vi "rsscope_core_global.vi"() -> ()   [LabVIEW 2014] (continued)
"Descriptive Name"="Trigger Event Beep", "Data Type"=0, "Command"="TRIG:EVEN:BEEP", "Access"=2, "Range Table"="RsScope_rngTriggerEvent", "Read Callback"="", "Write Callback"="", "Supported Models"="", "Instrument Options"="", "Flags"=0, "Help"="Generates a beep sound if the command is set to trigger.\n\nAvailable Repeated Capabilities:\nNone\n\nRemote-control command(s):\nTRIGger<m>:EVENt:BEEP"}, {"Level"=2, "Class Only"=FALSE, "Identifier"="RSSCOPE_ATTR_TRIGGER_EVENT_PRINT", "Descriptive Name"="Trigger Event Print", "Data Type"=0, "Command"="TRIG:EVEN:PRIN", "Access"=2, "Range Table"="RsScope_rngTriggerEvent", "Read Callback"="", "Write Callback"="", "Supported Models"="", "Instrument Options"="", "Flags"=0, "Help"="Saves a screenshot at each trigger if the command is set to trigger.\n\nAvailable Repeated Capabilities:\nNone\n\nRemote-control command(s):\nTRIGger<m>:EVENt:PRINt"}, {"Level"=2, "Class Only"=FALSE, "Identifier"="RSSCOPE_ATTR_TRIGGER_EVENT_SAVE_WAVEFORM", "Descriptive Name"="Trigger Event Save Waveform", "Data Type"=0, "Command"="TRIG:EVEN:WFMS", "Access"=2, "Range Table"="RsScope_rngTriggerEvent", "Read Callback"="", "Write Callback"="", "Supported Models"="", "Instrument Options"="", "Flags"=0, "Help"="Saves the waveform data to file at each trigger if the command is set to trigger.\n\nAvailable Repeated Capabilities:\nNone\n\nRemote-control command(s):\nTRIGger<m>:EVENt:WFMSave"}, {"Level"=2, "Class Only"=FALSE, "Identifier"="RSSCOPE_ATTR_TRIGGER_EVENT_RUN_EXTERNAL_APPLICATION", "Descriptive Name"="Trigger Event Run External Application", "Data Type"=0, "Command"="TRIG:EVEN:RUN", "Access"=2, "Range Table"="RsScope_rngTriggerEvent", "Read Callback"="", "Write Callback"="", "Supported Models"="", "Instrument Options"="", "Flags"=0, "Help"="Starts an external application if the attribute is set to trigger.\nUse the following attributes to set up the application:\nRSSCOPE_ATTR_EXTERNAL_APPLICATION_NAME\nRSSCOPE_ATTR_EXTERNAL_APPLICATION_PARAMETER\nRSSCOPE_ATTR_EXTERNAL_APPLICATION_WORKING_DIRECTORY\n\nAvailable Repeated Capabilities:\nNone\n\nRemote-control command(s):\nTRIGger<m>:EVENt:RUNexec"}, {"Level"=2, "Class Only"=FALSE, "Identifier"="RSSCOPE_ATTR_TRIGGER_EXTERNAL_OVERLOAD", "Descriptive Name"="Trigger External Overload", "Data Type"=3, "Command"="TRIG{Trigger}:EXT:OVER", "Access"=2, "Range Table"="", "Read Callback"="", "Write Callback"="", "Supported Models"="", "Instrument Options"="", "Flags"=0, "Help"="Sets the overload status of the external trigger input.\n\nAvailable Repeated Capabilities:\nTrigger: TrigA, TrigB, TrigR\r\n\nRemote-control command(s):\nTRIGger<m>:EXTern:OVERload"}, {"Level"=2, "Class Only"=FALSE, "Identifier"="RSSCOPE_ATTR_DIGITAL_FILTER_TRIGGER_COUPLING", "Descriptive Name"="Digital Filter Trigger Coupling", "Data Type"=0, "Command"="TRIG{Trigger}:COUP", "Access"=2, "Range Table"="rsscope_rngDSPTriggCoupling", "Read Callback"="", "Write Callback"="", "Supported Models"="", "Instrument Options"="", "Flags"=0, "Help"="Selects the filter for the trigger channel(s). Other channels must use the same filter, or proceed unfiltered.\n\nAvailable Repeated Capabilities:\nTrigger: TrigA, TrigB, TrigR\r\n\nRemote-control command(s):\nTRIGger<m>:COUPling"}, {"Level"=2, "Class Only"=FALSE, "Identifier"="RSSCOPE_ATTR_HIGH_FREQUENCY_REJECT_TRIGGER_STATE", "Descriptive Name"="High Frequency Reject Trigger State", "Data Type"=3, "Command"="TRIG{Trigger}:RFSR", "Access"=2, "Range Table"="", "Read Callback"="", "Write Callback"="", "Supported Models"="RTE", "Instrument Options"="", "Flags"=0, "Help"="Enables the DSP filter for the trigger channel. Frequencies higher than the bandwidth (RSSCOPE_ATTR_DIGITAL_FILTER_TRIGGER_RF_REJECT) are rejected, lower frequencies pass the filter.\n\nAvailable Repeated Capabilities:\nTrigger: TrigA, TrigB, TrigR\r\n\nRemote-control command(s):\nTRIGger<m>:RFSReject"}, {"Level"=2, "Class Only"=FALSE, "Identifier"="RSSCOPE_ATTR_TRIGGER_AC_POWER_INPUT_SLOPE", "Descriptive Name"="Trigger AC Power Input Slope", "Data Type"=0, "Command"="TRIG{Trigger}:POW:SLOP", "Access"=2, "Range Table"="rsscope_rngTriggerACPowerInputSlope", "Read Callback"="", "Write Callback"="", "Supported Models"="RTE", "Instrument Options"="", "Flags"=0, "Help"="Selects the rising or falling edges of the AC power input for the trigger condition.\n\nAvailable Repeated Capabilities:\nTrigger: TrigA, TrigB, TrigR\r\n\nRemote-control command(s):\nTRIGger<m>:POWerline:SLOPe"}, {"Level"=2, "Class Only"=TRUE, "Identifier"="", "Descriptive Name"="Channel", "Data Type"=0, "Command"="", "Access"=0, "Range Table"="", "Read Callback"="", "Write Callback"="", "Supported Models"="", "Instrument Options"="", "Flags"=0, "Help"="Indicates the trigger source channel"}, {"Level"=3, "Class Only"=FALSE, "Identifier"="RSSCOPE_ATTR_TRIGGER_LEVEL", "Descriptive Name"="Trigger Level", "Data Type"=1, "Command"="TRIG{Trigger}:LEV{TriggerSource}", "Access"=2, "Range Table"="", "Read Callback"="", "Write Callback"="", "Supported Models"="", "Instrument Options"="", "Flags"=0, "Help"="Sets the trigger level for the specified event and source.\n\nAvailable Repeated Capabilities:\nTrigger: TrigA, TrigB, TrigR\r\nTriggerSource: TsCH1, TsCH2, TsCH3, TsCH4, TsExt, TsLine, TsZ1V1, TsZ1V2, TsZ1V3, TsZ1V4, TsZ1I1, TsZ1I2, TsZ1I3, TsZ1I4, TsZ2V1, TsZ2V2, TsZ2V3, TsZ2V4, TsZ2I1, TsZ2I2, TsZ2I3, TsZ2I4, TsDiff1, TsDiff2, TsCommon1, TsCommon2\r\n\nRemote-control command(s):\nTRIGger<m>:LEVel<n>[:VALue]"}, {"Level"=3, "Class Only"=FALSE, "Identifier"="RSSCOPE_ATTR_DIGITAL_FILTER_TRIGGER_RF_REJECT", "Descriptive Name"="Digital Filter Trigger RF Reject", "Data Type"=1, "Command"="TRIG{Trigger}:RFR", "Access"=2, "Range Table"="rsscope_rngDSPTriggRFReject", "Read Callback"="", "Write Callback"="", "Supported Models"="", "Instrument Options"="", "Flags"=0, "Help"="Sets the limit frequency, if the trigger coupling is set to RFReject. See RSSCOPE_ATTR_DIGITAL_FILTER_TRIGGER_COUPLING\n\nAvailable Repeated Capabilities:\nTrigger: TrigA, TrigB, TrigR\r\n\nRemote-control command(s):\nTRIGger<m>:RFReject"}, {"Level"=2, "Class Only"=TRUE, "Identifier"="", "Descriptive Name"="Edge Triggering", "Data Type"=0, "Command"="", "Access"=0, "Range Table"="", "Read Callback"="", "Write Callback"="", "Supported Models"="", "Instrument Options"="", "Flags"=0, "Help"="Attributes that configure the edge trigger.  An edge trigger occurs when the trigger signal passes through the voltage threshold you specify with the RSSCOPE_ATTR_TRIGGER_LEVEL attribute and has the slope you specify with the RSSCOPE_ATTR_TRIGGER_SLOPE attribute."}, {"Level"=3, "Class Only"=FALSE, "Identifier"="RSSCOPE_ATTR_EXTERNAL_TRIGGER_COUPLING", "Descriptive Name"="External Trigger Coupling", "Data Type"=0, "Command"="TRIG:ANED:COUP", "Access"=2, "Range Table"="rsscope_rngTriggerCoupling", "Read Callback"="", "Write Callback"="", "Supported Models"="", "Instrument Options"="", "Flags"=0, "Help"="Sets the coupling for the analog trigger signal.\n\nAvailable Repeated Capabilities:\nNone\n\nRemote-control command(s):\nTRIGger<m>:ANEDge:COUPling"}, {"Level"=3, "Class Only"=FALSE, "Identifier"="RSSCOPE_ATTR_TRIGGER_SLOPE", "Descriptive Name"="Trigger Slope", "Data Type"=0, "Command"="TRIG{Trigger}:EDGE:SLOP", "Access"=2, "Range Table"="rsscope_rngTriggerSlope", "Read Callback"="", "Write Callback"="", "Supported Models"="", "Instrument Options"="", "Flags"=0, "Help"="Sets the slope for the edge trigger.\n\nAvailable Repeated Capabilities:\nTrigger: TrigA, TrigB, TrigR\r\n\nRemote-control command(s):\nTRIGger<m>:EDGE:SLOPe"}, {"Level"=3, "Class Only"=FALSE, "Identifier"="RSSCOPE_ATTR_EXTERNAL_TRIGGER_LEVEL", "Descriptive Name"="External Trigger Level", "Data Type"=1, "Command"="TRIG:LEV5", "Access"=2, "Range Table"="", "Read Callback"="", "Write Callback"="", "Supported Models"="", "Instrument Options"="", "Flags"=0, "Help"="Sets the trigger level for the analog external trigger input.\n\nAvailable Repeated Capabilities:\nNone\n\nRemote-control command(s):\nTRIGger<m>:LEVel<n>[:VALue]"}, {"Level"=3, "Class Only"=FALSE, "Identifier"="RSSCOPE_ATTR_EXTERNAL_TRIGGER_FILTER_CUT_OFF_FREQUENCY_HIGHPASS", "Descriptive Name"="External Trigger Filter Cut Off Frequency Highpass", "Data Type"=0, "Command"="TRIG:ANED:CUT:HIGH", "Access"=2, "Range Table"="rsscope_rngCutOffFrequency", "Read Callback"="", "Write Callback"="", "Supported Models"="", "Instrument Options"="", "Flags"=0, "Help"="Defines highpass &apos;Cut-off&apos; frequency of filter.\n\nAvailable Repeated Capabilities:\nNone\n\nRemote-control command(s):\nTRIGger<m>:ANEDge:CUToff:HIGHpass"}, {"Level"=3, "Class Only"=FALSE, "Identifier"="RSSCOPE_ATTR_EXTERNAL_TRIGGER_FILTER_CUT_OFF_FREQUENCY_LOWPASS", "Descriptive Name"="External Trigger Filter Cut Off Frequency Lowpass", "Data Type"=0, "Command"="TRIGger1:ANED:CUT:LOWP", "Access"=2, "Range Table"="rsscope_rngCutOffFrequency", "Read Callback"="", "Write Callback"="", "Supported Models"="", "Instrument Options"="", "Flags"=0, "Help"="Defines lowpass &apos;Cut-off&apos; frequency of filter.\n\nAvailable Repeated Capabilities:\nNone\n\nRemote-control command(s):\nTRIGger<m>:ANEDge:CUToff:LOWPass"}, {"Level"=3, "Class Only"=FALSE, "Identifier"="RSSCOPE_ATTR_EXTERNAL_TRIGGER_FILTER", "Descriptive Name"="External Trigger Filter", "Data Type"=0, "Command"="TRIG:ANED:FILT", "Access"=2, "Range Table"="rsscope_rngFilterType", "Read Callback"="", "Write Callback"="", "Supported Models"="", "Instrument Options"="", "Flags"=0, "Help"="The analog trigger signal is used for triggering; you can directly select an additional filter to reject high or low frequencies.\n\nAvailable Repeated Capabilities:\nNone\n\nRemote-control command(s):\nTRIGger<m>:ANEDge:FILTer"}, {"Level"=3, "Class Only"=FALSE, "Identifier"="RSSCOPE_ATTR_EXTERNAL_TRIGGER_GROUND_CONNECTION_ENABLED", "Descriptive Name"="External Trigger Ground Connection Enabled", "Data Type"=3, "Command"="TRIG:ANED:GND", "Access"=2, "Range Table"="", "Read Callback"="", "Write Callback"="", "Supported Models"="", "Instrument Options"="", "Flags"=0, "Help"="Connects the analog signal to the ground.\n\nAvailable Repeated Capabilities:\nNone\n\nRemote-control command(s):\nTRIGger<m>:ANEDge:GND"}, {"Level"=3, "Class Only"=FALSE, "Identifier"="RSSCOPE_ATTR_EXTERNAL_TRIGGER_SLOPE", "Descriptive Name"="External Trigger Slope", "Data Type"=0, "Command"="TRIG:ANED:SLOP", "Access"=2, "Range Table"="rsscope_rngPolarity", "Read Callback"="", "Write Callback"="", "Supported Models"="", "Instrument Options"="", "Flags"=0, "Help"="Sets the edge for the trigger event. Value 'Either' is not allowed.\n\nAvailable Repeated Capabilities:\nNone\n\nRemote-control command(s):\nTRIGger<m>:ANEDge:SLOPe"}, {"Level"=3, "Class Only"=FALSE, "Identifier"="RSSCOPE_ATTR_EXTERNAL_TRIGGER_NOISE_REJECT", "Descriptive Name"="External Trigger Noise Reject", "Data Type"=3, "Command"="TRIGger1:ANED:NREJ", "Access"=2, "Range Table"="", "Read Callback"="", "Write Callback"="", "Supported Models"="", "Instrument Options"="", "Flags"=0, "Help"="Enables/disbales the noise reject for the external trigger input.\n\nAvailable Repeated Capabilities:\nNone\n\nRemote-control command(s):\nTRIGger<m>:ANEDge:NREJect"}, {"Level"=2, "Class Only"=TRUE, "Identifier"="", "Descriptive Name"="Runt Triggering", "Data Type"=0, "Command"="", "Access"=0, "Range Table"="", "Read Callback"="", "Write Callback"="", "Supported Models"="", "Instrument Options"="", "Flags"=0, "Help"="A runt is a pulse lower than normal in amplitude. The amplitude crosses the first threshold twice in succession without crossing the second one. In addition to the threshold amplitudes, you can define a time limit for the runt in the same way as for width triggers. For example, this trigger can detect logic, digital, and analog signals remaining below a specified threshold amplitude because I/O ports are in undefined state."}, {"Level"=3, "Class Only"=FALSE, "Identifier"="RSSCOPE_ATTR_RUNT_CONDITION", "Descriptive Name"="Runt Condition", "Data Type"=0, "Command"="TRIG{Trigger}:RUNT:RANG", "Access"=2, "Range Table"="rsscope_rngRuntCondition", "Read Callback"="", "Write Callback"="", "Supported Models"="", "Instrument Options"="", "Flags"=0, "Help"="Defines the time limit of the runt pulse in relation to the TRIGger<m>: RUNT: WIDTh and TRIGger<m>: RUNT: DELTa settings.\n\nAvailable Repeated Capabilities:\nTrigger: TrigA, TrigB, TrigR\r\n\nRemote-control command(s):\nTRIGger<m>:RUNT:RANGe"}, {"Level"=3, "Class Only"=FALSE, "Identifier"="RSSCOPE_ATTR_RUNT_WIDTH", "Descriptive Name"="Runt Width", "Data Type"=1, "Command"="TRIG{Trigger}:RUNT:WIDT", "Access"=2, "Range Table"="rsscope_rngWidth", "Read Callback"="", "Write Callback"="", "Supported Models"="", "Instrument Options"="", "Flags"=0, "Help"="Defines the upper or lower voltage threshold.\n\nAvailable Repeated Capabilities:\nTrigger: TrigA, TrigB, TrigR\r\n\nRemote-control command(s):\nTRIGger<m>:RUNT:WIDTh"}, {"Level"=3, "Class Only"=FALSE, "Identifier"="RSSCOPE_ATTR_RUNT_DELTA", "Descriptive Name"="Runt Delta", "Data Type"=1, "Command"="TRIG{Trigger}:RUNT:DELT", "Access"=2, "Range Table"="", "Read Callback"="", "Write Callback"="", "Supported Models"="", "Instrument Options"="", "Flags"=0, "Help"="Defines a range around the runt width specified using TRIGger<m>: RUNT: WIDTh. This attribute is only available if TRIGger<m>: RUNT: RANGe is set to &apos;WITHin&apos; or &apos;OUTSide&apos;\n\nAvailable Repeated Capabilities:\nTrigger: TrigA, TrigB, TrigR\r\n\nRemote-control command(s):\nTRIGger<m>:RUNT:DELTa"}, {"Level"=3, "Class Only"=FALSE, "Identifier"="RSSCOPE_ATTR_RUNT_POLARITY", "Descriptive Name"="Runt Polarity", "Data Type"=0, "Command"="TRIG{Trigger}:RUNT:POL", "Access"=2, "Range Table"="rsscope_rngTriggerSlope", "Read Callback"="", "Write Callback"="", "Supported Models"="", "Instrument Options"="", "Flags"=0, "Help"="Defines the polarity of a pulse, that is the direction of the first pulse slope.\n\nAvailable Repeated Capabilities:\nTrigger: TrigA, TrigB, TrigR\r\n\nRemote-control command(s):\nTRIGger<m>:RUNT:POLarity"}, {"Level"=3, "Class Only"=TRUE, "Identifier"="", "Descriptive Name"="Trigger Source", "Data Type"=0, "Command"="", "Access"=0, "Range Table"="", "Read Callback"="", "Write Callback"="", "Supported Models"="", "Instrument Options"="", "Flags"=0, "Help"="Selects Trigger Source"}, {"Level"=4, "Class Only"=FALSE, "Identifier"="RSSCOPE_ATTR_RUNT_HIGH_THRESHOLD", "Descriptive Name"="Runt High Threshold", "Data Type"=1, "Command"="TRIG{Trigger}:LEV{TriggerSource}:RUNT:UPP", "Access"=2, "Range Table"="", "Read Callback"="", "Write Callback"="", "Supported Models"="", "Instrument Options"="", "Flags"=0, "Help"="Sets the upper voltage threshold.\n\nAvailable Repeated Capabilities:\nTrigger: TrigA, TrigB, TrigR\r\nTriggerSource: TsCH1, TsCH2, TsCH3, TsCH4, TsExt, TsLine, TsZ1V1, TsZ1V2, TsZ1V3, TsZ1V4, TsZ1I1, TsZ1I2, TsZ1I3, TsZ1I4, TsZ2V1, TsZ2V2, TsZ2V3, TsZ2V4, TsZ2I1, TsZ2I2, TsZ2I3, TsZ2I4, TsDiff1, TsDiff2, TsCommon1, TsCommon2\r\n\nRemote-control command(s):\nTRIGger<m>:LEVel<n>:RUNT:UPPer"}, {"Level"=4, "Class Only"=FALSE, "Identifier"="RSSCOPE_ATTR_RUNT_LOW_THRESHOLD", "Descriptive Name"="Runt Low Threshold", "Data Type"=1, "Command"="TRIG{Trigger}:LEV{TriggerSource}:RUNT:LOW", "Access"=2, "Range Table"="", "Read Callback"="", "Write Callback"="", "Supported Models"="", "Instrument Options"="", "Flags"=0, "Help"="Sets the lower voltage threshold.\n\nAvailable Repeated Capabilities:\nTrigger: TrigA, TrigB, TrigR\r\nTriggerSource: TsCH1, TsCH2, TsCH3, TsCH4, TsExt, TsLine, TsZ1V1, TsZ1V2, TsZ1V3, TsZ1V4, TsZ1I1, TsZ1I2, TsZ1I3, TsZ1I4, TsZ2V1, TsZ2V2, TsZ2V3, TsZ2V4, TsZ2I1, TsZ2I2, TsZ2I3, TsZ2I4, TsDiff1, TsDiff2, TsCommon1, TsCommon2\r\n\nRemote-control command(s):\nTRIGger<m>:LEVel<n>:RUNT:LOWer"}, {"Level"=2, "Class Only"=TRUE, "Identifier"="", "Descriptive Name"="Glitch Triggering", "Data Type"=0, "Command"="", "Access"=0, "Range Table"="", "Read Callback"="", "Write Callback"="", "Supported Models"="", "Instrument Options"="", "Flags"=0, "Help"="The glitch trigger event detects pulses shorter or longer than a specified time. It identifies deviation from the nominal data rate and helps to analyze causes of even rare glitches and their effects on other signals."}, {"Level"=3, "Class Only"=FALSE, "Identifier"="RSSCOPE_ATTR_GLITCH_WIDTH", "Descriptive Name"="Glitch Width", "Data Type"=1, "Command"="TRIG{Trigger}:GLIT:WIDT", "Access"=2, "Range Table"="rsscope_rngWidth", "Read Callback"="", "Write Callback"="", "Supported Models"="", "Instrument Options"="", "Flags"=0, "Help"="Sets the length of a glitch. The instrument triggers on pulses shorter or longer than this value.\n\nAvailable Repeated Capabilities:\nTrigger: TrigA, TrigB, TrigR\r\n\nRemote-control command(s):\nTRIGger<m>:GLITch:WIDTh"}, {"Level"=3, "Class Only"=FALSE, "Identifier"="RSSCOPE_ATTR_GLITCH_POLARITY", "Descriptive Name"="Glitch Polarity", "Data Type"=0, "Command"="TRIG{Trigger}:GLIT:POL", "Access"=2, "Range Table"="rsscope_rngTriggerSlope", "Read Callback"="", "Write Callback"="", "Supported Models"="", "Instrument Options"="", "Flags"=0, "Help"="Defines the polarity of a pulse, that is the direction of the first pulse slope.\n\nAvailable Repeated Capabilities:\nTrigger: TrigA, TrigB, TrigR\r\n\nRemote-control command(s):\nTRIGger<m>:GLITch:POLarity"}, {"Level"=3, "Class Only"=FALSE, "Identifier"="RSSCOPE_ATTR_GLITCH_CONDITION", "Descriptive Name"="Glitch Condition", "Data Type"=0, "Command"="TRIG{Trigger}:GLIT:RANG", "Access"=2, "Range Table"="rsscope_rngGlitchCondition", "Read Callback"="", "Write Callback"="", "Supported Models"="", "Instrument Options"="", "Flags"=0, "Help"="Selects which glitches are identified: shorter or longer than the width.\n\nAvailable Repeated Capabilities:\nTrigger: TrigA, TrigB, TrigR\r\n\nRemote-control command(s):\nTRIGger<m>:GLITch:RANGe"}, {"Level"=2, "Class Only"=TRUE, "Identifier"="", "Descriptive Name"="Width Triggering", "Data Type"=0, "Command"="", "Access"=0, "Range Table"="", "Read Callback"="", "Write Callback"="", "Supported Models"="", "Instrument Options"="", "Flags"=0, "Help"="Attributes that configure the oscilloscope for width triggering.  You use these attributes to configure the oscilloscope after you set the RSSCOPE_ATTR_TRIGGER_TYPE to RSSCOPE_VAL_WIDTH_TRIGGER.\nA width trigger occurs when the oscilloscope detects a positive or negative pulse with a width between, or optionally outside, the width thresholds. The trigger occurs when the edge of a pulse that corresponds to the width thresholds, width condition, and polarity you specify crosses the trigger level you specify with the RSSCOPE_ATTR_TRIGGER_LEVEL attribute."}, {"Level"=3, "Class Only"=FALSE, "Identifier"="RSSCOPE_ATTR_WIDTH_CONDITION", "Descriptive Name"="Width Condition", "Data Type"=0, "Command"="TRIG{Trigger}:WIDT:RANG", "Access"=2, "Range Table"="rsscope_rngWidthCondition", "Read Callback"="", "Write Callback"="", "Supported Models"="", "Instrument Options"="", "Flags"=0, "Help"="Sets how the measured pulse width is compared with the given limit(s).\n\nAvailable Repeated Capabilities:\nTrigger: TrigA, TrigB, TrigR\r\n\nRemote-control command(s):\nTRIGger<m>:WIDTh:RANGe"}, {"Level"=3, "Class Only"=FALSE, "Identifier"="RSSCOPE_ATTR_WIDTH", "Descriptive Name"="Width", "Data Type"=1, "Command"="TRIG{Trigger}:WIDT:WIDT", "Access"=2, "Range Table"="", "Read Callback"="", "Write Callback"="", "Supported Models"="", "Instrument Options"="", "Flags"=0, "Help"="For the ranges &apos;Within&apos; and &apos;Outside&apos;, the width defines the center of a range which is defined by the limits &apos;+/-Delta&apos;. For the ranges &apos;Shorter&apos; and &apos;Longer&apos;, the width defines the maximum and minimum pulse width, respectively.\n\nAvailable Repeated Capabilities:\nTrigger: TrigA, TrigB, TrigR\r\n\nRemote-control command(s):\nTRIGger<m>:WIDTh:WIDTh"}, {"Level"=3, "Class Only"=FALSE, "Identifier"="RSSCOPE_ATTR_WIDTH_DELTA", "Descriptive Name"="Width Delta", "Data Type"=1, "Command"="TRIG{Trigger}:WIDT:DELT", "Access"=2, "Range Table"="", "Read Callback"="", "Write Callback"="", "Supported Models"="", "Instrument Options"="", "Flags"=0, "Help"="Defines a range around the width value.\n\nAvailable Repeated Capabilities:\nTrigger: TrigA, TrigB, TrigR\r\n\nRemote-control command(s):\nTRIGger<m>:WIDTh:DELTa"}, {"Level"=3, "Class Only"=FALSE, "Identifier"="RSSCOPE_ATTR_WIDTH_POLARITY", "Descriptive Name"="Width Polarity", "Data Type"=0, "Command"="TRIG{Trigger}:WIDT:POL", "Access"=2, "Range Table"="rsscope_rngPolarity", "Read Callback"="", "Write Callback"="", "Supported Models"="", "Instrument Options"="", "Flags"=0, "Help"="Sets the polarity of the pulse.\n\nAvailable Repeated Capabilities:\nTrigger: TrigA, TrigB, TrigR\r\n\nRemote-control command(s):\nTRIGger<m>:WIDTh:POLarity"}, {"Level"=2, "Class Only"=TRUE, "Identifier"="", "Descriptive Name"="Window Triggering", "Data Type"=0, "Command"="", "Access"=0, "Range Table"="", "Read Callback"="", "Write Callback"="", "Supported Models"="", "Instrument Options"="", "Flags"=0, "Help"="The window trigger checks the signal run in relation to a &apos;window&apos;. The window is formed by the upper and lower voltage levels. The event condition is fulfilled, if the waveform enters or leaves the window, or if the waveform stays inside or outside for a time longer or shorter than specified. With the window trigger, you can display longer transient effects."}, {"Level"=3, "Class Only"=FALSE, "Identifier"="RSSCOPE_ATTR_WINDOW_CONDITION", "Descriptive Name"="Window Condition", "Data Type"=0, "Command"="TRIG{Trigger}:WIND:RANG", "Access"=2, "Range Table"="rsscope_rngWindowCondition", "Read Callback"="", "Write Callback"="", "Supported Models"="", "Instrument Options"="", "Flags"=0, "Help"="Defines the signal run in relation to the window.\n\nAvailable Repeated Capabilities:\nTrigger: TrigA, TrigB, TrigR\r\n\nRemote-control command(s):\nTRIGger<m>:WINDow:RANGe"}, {"Level"=3, "Class Only"=FALSE, "Identifier"="RSSCOPE_ATTR_WINDOW_WIDTH", "Descriptive Name"="Window Width", "Data Type"=1, "Command"="TRIG{Trigger}:WIND:WIDT", "Access"=2, "Range Table"="rsscope_rngWidth", "Read Callback"="", "Write Callback"="", "Supported Models"="", "Instrument Options"="", "Flags"=0, "Help"="For the ranges &apos;Within&apos; and &apos;Outside&apos;, the width defines the center of a time range which is defined by the limits &apos;Delta&apos;.\nFor the ranges &apos;Shorter&apos; and &apos;Longer&apos;, it defines the maximum and minimum time lapse, respectively.\n\nAvailable Repeated Capabilities:\nTrigger: TrigA, TrigB, TrigR\r\n\nRemote-control command(s):\nTRIGger<m>:WINDow:WIDTh"}, {"Level"=3, "Class Only"=FALSE, "Identifier"="RSSCOPE_ATTR_WINDOW_DELTA", "Descriptive Name"="Window Delta", "Data Type"=1, "Command"="TRIG{Trigger}:WIND:DELT", "Access"=2, "Range Table"="", "Read Callback"="", "Write Callback"="", "Supported Models"="", "Instrument Options"="", "Flags"=0, "Help"="Defines a range around the &apos;Width&apos; value.\n\nAvailable Repeated Capabilities:\nTrigger: TrigA, TrigB, TrigR\r\n\nRemote-control command(s):\nTRIGger<m>:WINDow:DELTa"}, {"Level"=3, "Class Only"=FALSE, "Identifier"="RSSCOPE_ATTR_WINDOW_TIME_CONDITION", "Descriptive Name"="Window Time Condition", "Data Type"=0, "Command"="TRIG{Trigger}:WIND:TIME", "Access"=2, "Range Table"="rsscope_rngWidthCondition", "Read Callback"="", "Write Callback"="", "Supported Models"="", "Instrument Options"="", "Flags"=0, "Help"="Selects how the time limit of the window is defined. Time conditioning is available for the vertical conditions &apos;Stay within&apos; and &apos;Stay outside&apos;.\n\nAvailable Repeated Capabilities:\nTrigger: TrigA, TrigB, TrigR\r\n\nRemote-control command(s):\nTRIGger<m>:WINDow:TIME"}, {"Level"=3, "Class Only"=TRUE, "Identifier"="", "Descriptive Name"="Trigger Source", "Data Type"=0, "Command"="", "Access"=0, "Range Table"="", "Read Callback"="", "Write Callback"="", "Supported Models"="", "Instrument Options"="", "Flags"=0, "Help"="Selects Trigger Source"}, {"Level"=4, "Class Only"=FALSE, "Identifier"="RSSCOPE_ATTR_WINDOW_UPPER_LIMIT", "Descriptive Name"="Window Upper Limit", "Data Type"=1, "Command"="TRIG{Trigger}:LEV{TriggerSource}:WIND:UPP", "Access"=2, "Range Table"="", "Read Callback"="", "Write Callback"="", "Supported Models"="", "Instrument Options"="", "Flags"=0, "Help"="Sets the upper voltage limit for the window.\n\nAvailable Repeated Capabilities:\nTrigger: TrigA, TrigB, TrigR\r\nTriggerSource: TsCH1, TsCH2, TsCH3, TsCH4, TsExt, TsLine, TsZ1V1, TsZ1V2, TsZ1V3, TsZ1V4, TsZ1I1, TsZ1I2, TsZ1I3, TsZ1I4, TsZ2V1, TsZ2V2, TsZ2V3, TsZ2V4, TsZ2I1, TsZ2I2, TsZ2I3, TsZ2I4, TsDiff1, TsDiff2, TsCommon1, TsCommon2\r\n\nRemote-control command(s):\nTRIGger<m>:LEVel<n>:WINDow:UPPer"}, {"Level"=4, "Class Only"=FALSE, "Identifier"="RSSCOPE_ATTR_WINDOW_LOWER_LIMIT", "Descriptive Name"="Window Lower Limit", "Data Type"=1, "Command"="TRIG{Trigger}:LEV{TriggerSource}:WIND:LOW", "Access"=2, "Range Table"="", "Read Callback"="", "Write Callback"="", "Supported Models"="", "Instrument Options"="", "Flags"=0, "Help"="Sets the lower voltage limit for the window.\n\nAvailable Repeated Capabilities:\nTrigger: TrigA, TrigB, TrigR\r\nTriggerSource: TsCH1, TsCH2, TsCH3, TsCH4, TsExt, TsLine, TsZ1V1, TsZ1V2, TsZ1V3, TsZ1V4, TsZ1I1, TsZ1I2, TsZ1I3, TsZ1I4, TsZ2V1, TsZ2V2, TsZ2V3, TsZ2V4, TsZ2I1, TsZ2I2, TsZ2I3, TsZ2I4, TsDiff1, TsDiff2, TsCommon1, TsCommon2\r\n\nRemote-control command(s):\nTRIGger<m>:LEVel<n>:WINDow:LOWer"}, {"Level"=2, "Class Only"=TRUE, "Identifier"="", "Descriptive Name"="Timeout Triggering", "Data Type"=0, "Command"="", "Access"=0, "Range Table"="", "Read Callback"="", "Write Callback"="", "Supported Models"="", "Instrument Options"="", "Flags"=0, "Help"="The timeout trigger event checks if the signal stays above or below the threshold voltage for a specified time lapse. In other words, the event occurs if the trigger source does not have the expected transition within the specified time."}, {"Level"=3, "Class Only"=FALSE, "Identifier"="RSSCOPE_ATTR_TIMEOUT_CONDITION", "Descriptive Name"="Timeout Condition", "Data Type"=0, "Command"="TRIG{Trigger}:TIMeout:RANG", "Access"=2, "Range Table"="rsscope_rngTimeoutCondition", "Read Callback"="", "Write Callback"="", "Supported Models"="", "Instrument Options"="", "Flags"=0, "Help"="Defines the relation of the signal level to the trigger level.\n\nAvailable Repeated Capabilities:\nTrigger: TrigA, TrigB, TrigR\r\n\nRemote-control command(s):\nTRIGger<m>:TIMeout:RANGe"}, {"Level"=3, "Class Only"=FALSE, "Identifier"="RSSCOPE_ATTR_TIMEOUT_VALUE", "Descriptive Name"="Timeout Value", "Data Type"=1, "Command"="TRIG{Trigger}:TIMeout:TIME", "Access"=2, "Range Table"="rsscope_rngWidth", "Read Callback"="", "Write Callback"="", "Supported Models"="", "Instrument Options"="", "Flags"=0, "Help"="Defines the time limit for the timeout at which the instrument triggers.\n\nAvailable Repeated Capabilities:\nTrigger: TrigA, TrigB, TrigR\r\n\nRemote-control command(s):\nTRIGger<m>:TIMeout:TIME"}, {"Level"=2, "Class Only"=TRUE, "Identifier"="", "Descriptive Name"="Interval Triggering", "Data Type"=0, "Command"="", "Access"=0, "Range Table"="", "Read Callback"="", "Write Callback"="", "Supported Models"="", "Instrument Options"="", "Flags"=0, "Help"="The interval trigger analyzes the time between two pulses. While the interval trigger can only analyze either positive or negative polarity, searching for an interval is also possible for both polarities at the same time (&apos;Either&apos;)."}, {"Level"=3, "Class Only"=FALSE, "Identifier"="RSSCOPE_ATTR_INTERVAL_CONDITION", "Descriptive Name"="Interval Condition", "Data Type"=0, "Command"="TRIG{Trigger}:INT:RANG", "Access"=2, "Range Table"="rsscope_rngWidthCondition", "Read Callback"="", "Write Callback"="", "Supported Models"="", "Instrument Options"="", "Flags"=0, "Help"="Defines the range of an interval in relation to the interval width.\n\nAvailable Repeated Capabilities:\nTrigger: TrigA, TrigB, TrigR\r\n\nRemote-control command(s):\nTRIGger<m>:INTerval:RANGe"}, {"Level"=3, "Class Only"=FALSE, "Identifier"="RSSCOPE_ATTR_INTERVAL_WIDTH", "Descriptive Name"="Interval Width", "Data Type"=1, "Command"="TRIG{Trigger}:INT:WIDT", "Access"=2, "Range Table"="rsscope_rngWidth", "Read Callback"="", "Write Callback"="", "Supported Models"="", "Instrument Options"="", "Flags"=0, "Help"="Defines the time between two pulses.\n\nAvailable Repeated Capabilities:\nTrigger: TrigA, TrigB, TrigR\r\n\nRemote-control command(s):\nTRIGger<m>:INTerval:WIDTh"}, {"Level"=3, "Class Only"=FALSE, "Identifier"="RSSCOPE_ATTR_INTERVAL_DELTA", "Descriptive Name"="Interval Delta", "Data Type"=1, "Command"="TRIG{Trigger}:INT:DELT", "Access"=2, "Range Table"="", "Read Callback"="", "Write Callback"="", "Supported Models"="", "Instrument Options"="", "Flags"=0, "Help"="Defines a range around the &apos;Interval width&apos; value.\n\nAvailable Repeated Capabilities:\nTrigger: TrigA, TrigB, TrigR\r\n\nRemote-control command(s):\nTRIGger<m>:INTerval:DELTa"}, {"Level"=3, "Class Only"=FALSE, "Identifier"="RSSCOPE_ATTR_INTERVAL_POLARITY", "Descriptive Name"="Interval Polarity", "Data Type"=0, "Command"="TRIG{Trigger}:INT:SLOP", "Access"=2, "Range Table"="rsscope_rngPolarity", "Read Callback"="", "Write Callback"="", "Supported Models"="", "Instrument Options"="", "Flags"=0, "Help"="Sets the edge for the trigger. You can analyze the interval between positive edges or between negative edges.\n\nAvailable Repeated Capabilities:\nTrigger: TrigA, TrigB, TrigR\r\n\nRemote-control command(s):\nTRIGger<m>:INTerval:SLOPe"}, {"Level"=2, "Class Only"=TRUE, "Identifier"="", "Descriptive Name"="Slew Rate Triggering", "Data Type"=0, "Command"="", "Access"=0, "Range Table"="", "Read Callback"="", "Write Callback"="", "Supported Models"="", "Instrument Options"="", "Flags"=0, "Help"="The slew rate trigger, also known as transition trigger, can detect fast or slow edges selectively. It triggers on edges, if the transition time from the lower to higher voltage level (or vice versa) is shorter or longer as defined, or outside a specified time range. The trigger event finds slew rates faster than expected or permissible to avoid overshooting and other interfering effects. It also detects very slow edges violating the timing in pulse series.\n\nThe slew rate trigger is not available for the B-event (Suffix = 2)."}, {"Level"=3, "Class Only"=FALSE, "Identifier"="RSSCOPE_ATTR_SLEW_CONDITION", "Descriptive Name"="Slew Condition", "Data Type"=0, "Command"="TRIG{Trigger}:SLEW:RANG", "Access"=2, "Range Table"="rsscope_rngSlewCondition", "Read Callback"="", "Write Callback"="", "Supported Models"="", "Instrument Options"="", "Flags"=0, "Help"="Defines the time limit for the slew rate in relation to the upper or lower trigger level. The time measurement starts when the signal crosses the first trigger level - the upper or lower level depending on the selected slope - and stops when the signal crosses the second level.\n\nAvailable Repeated Capabilities:\nTrigger: TrigA, TrigB, TrigR\r\n\nRemote-control command(s):\nTRIGger<m>:SLEW:RANGe"}, {"Level"=3, "Class Only"=FALSE, "Identifier"="RSSCOPE_ATTR_SLEW_RATE", "Descriptive Name"="Slew Rate", "Data Type"=1, "Command"="TRIG{Trigger}:SLEW:RATE", "Access"=2, "Range Table"="rsscope_rngWidth", "Read Callback"="", "Write Callback"="", "Supported Models"="", "Instrument Options"="", "Flags"=0, "Help"="For the ranges &apos;Within&apos; and &apos;Outside&apos;, the slew rate defines the center of a range which is defined by the limits &apos;Delta&apos;.\nFor the ranges &apos;Shorter&apos; and &apos;Longer&apos;, the slew rate defines the maximum and minimum slew rate limits, respectively. When the signal crosses this level, the slew rate measurement starts or stops depending on the selected slope.\n\nAvailable Repeated Capabilities:\nTrigger: TrigA, TrigB, TrigR\r\n\nRemote-control command(s):\nTRIGger<m>:SLEW:RATE"}, {"Level"=3, "Class Only"=FALSE, "Identifier"="RSSCOPE_ATTR_SLEW_DELTA", "Descriptive Name"="Slew Delta", "Data Type"=1, "Command"="TRIG{Trigger}:SLEW:DELT", "Access"=2, "Range Table"="", "Read Callback"="", "Write Callback"="", "Supported Models"="", "Instrument Options"="", "Flags"=0, "Help"="Defines a time range around the slew rate.\n\nAvailable Repeated Capabilities:\nTrigger: TrigA, TrigB, TrigR\r\n\nRemote-control command(s):\nTRIGger<m>:SLEW:DELTa"}, {"Level"=3, "Class Only"=FALSE, "Identifier"="RSSCOPE_ATTR_SLEW_POLARITY", "Descriptive Name"="Slew Polarity", "Data Type"=0, "Command"="TRIG{Trigger}:SLEW:SLOP", "Access"=2, "Range Table"="rsscope_rngPolarity", "Read Callback"="", "Write Callback"="", "Supported Models"="", "Instrument Options"="", "Flags"=0, "Help"="Selects the edge type for the trigger event.\n\nAvailable Repeated Capabilities:\nTrigger: TrigA, TrigB, TrigR\r\n\nRemote-control command(s):\nTRIGger<m>:SLEW:SLOPe"}, {"Level"=3, "Class Only"=TRUE, "Identifier"="", "Descriptive Name"="Trigger Source", "Data Type"=0, "Command"="", "Access"=0, "Range Table"="", "Read Callback"="", "Write Callback"="", "Supported Models"="", "Instrument Options"="", "Flags"=0, "Help"="Selects Trigger Source"}, {"Level"=4, "Class Only"=FALSE, "Identifier"="RSSCOPE_ATTR_SLEW_UPPER_LIMIT", "Descriptive Name"="Slew Upper Limit", "Data Type"=1, "Command"="TRIG{Trigger}:LEV{TriggerSource}:SLEW:UPP", "Access"=2, "Range Table"="", "Read Callback"="", "Write Callback"="", "Supported Models"="", "Instrument Options"="", "Flags"=0, "Help"="Defines the upper voltage threshold. When the signal crosses this level, the slew rate measurement starts or stops depending on the selected slope.\n\nAvailable Repeated Capabilities:\nTrigger: TrigA, TrigB, TrigR\r\nTriggerSource: TsCH1, TsCH2, TsCH3, TsCH4, TsExt, TsLine, TsZ1V1, TsZ1V2, TsZ1V3, TsZ1V4, TsZ1I1, TsZ1I2, TsZ1I3, TsZ1I4, TsZ2V1, TsZ2V2, TsZ2V3, TsZ2V4, TsZ2I1, TsZ2I2, TsZ2I3, TsZ2I4, TsDiff1, TsDiff2, TsCommon1, TsCommon2\r\n\nRemote-control command(s):\nTRIGger<m>:LEVel<n>:SLEW:UPPer"}, {"Level"=4, "Class Only"=FALSE, "Identifier"="RSSCOPE_ATTR_SLEW_LOWER_LIMIT", "Descriptive Name"="Slew Lower Limit", "Data Type"=1, "Command"="TRIG{Trigger}:LEV{TriggerSource}:SLEW:LOW", "Access"=2, "Range Table"="", "Read Callback"="", "Write Callback"="", "Supported Models"="", "Instrument Options"="", "Flags"=0, "Help"="Defines the lower voltage threshold. When the signal crosses this level, the slew rate measurement starts or stops depending on the selected slope.\n\nAvailable Repeated Capabilities:\nTrigger: TrigA, TrigB, TrigR\r\nTriggerSource: TsCH1, TsCH2, TsCH3, TsCH4, TsExt, TsLine, TsZ1V1, TsZ1V2, TsZ1V3, TsZ1V4, TsZ1I1, TsZ1I2, TsZ1I3, TsZ1I4, TsZ2V1, TsZ2V2, TsZ2V3, TsZ2V4, TsZ2I1, TsZ2I2, TsZ2I3, TsZ2I4, TsDiff1, TsDiff2, TsCommon1, TsCommon2\r\n\nRemote-control command(s):\nTRIGger<m>:LEVel<n>:SLEW:LOWer"}, {"Level"=2, "Class Only"=TRUE, "Identifier"="", "Descriptive Name"="Data2Clock Triggering", "Data Type"=0, "Command"="", "Access"=0, "Range Table"="", "Read Callback"="", "Write Callback"="", "Supported Models"="", "Instrument Options"="", "Flags"=0, "Help"="With the Data2Clock event - also known as setup/hold - you can analyze the relative timing between two signals: a data signal and the synchronous clock signal. Many systems require, that the data signal must be steady for some time before and after the clock edge, for example, the data transmission on parallel interfaces. With this trigger type, you can also test the time correlation of sideband and inband signals. The event occurs if the data signal crosses the data level during the setup and hold time. The reference point for the time measurement is defined by clock level and clock edge.\n\nThe Data2Clock trigger is only available for the A-event (Suffix = 1)."}, {"Level"=3, "Class Only"=FALSE, "Identifier"="RSSCOPE_ATTR_DATA2CLOCK_SOURCE", "Descriptive Name"="Data2Clock Source", "Data Type"=0, "Command"="TRIG:SETH:CSO", "Access"=2, "Range Table"="rsscope_rngTriggerSourceChannelOnly", "Read Callback"="", "Write Callback"="", "Supported Models"="", "Instrument Options"="", "Flags"=0, "Help"="Selects the input channel of the clock signal.\n\nAvailable Repeated Capabilities:\nNone\n\nRemote-control command(s):\nTRIGger<m>:SETHold:CSOurce[:VALue]"}, {"Level"=3, "Class Only"=FALSE, "Identifier"="RSSCOPE_ATTR_DATA2CLOCK_LEVEL", "Descriptive Name"="Data2Clock Level", "Data Type"=1, "Command"="TRIG1:SETH:CSO:LEV", "Access"=2, "Range Table"="", "Read Callback"="", "Write Callback"="", "Supported Models"="", "Instrument Options"="", "Flags"=0, "Help"="Sets the voltage level for the clock signal. Both and RSSCOPE_ATTR_DATA2CLOCK_POLARITY define the starting point for calculation of the setup and hold time.\n\nAvailable Repeated Capabilities:\nNone\n\nRemote-control command(s):\nTRIGger<m>:SETHold:CSOurce:LEVel"}, {"Level"=3, "Class Only"=FALSE, "Identifier"="RSSCOPE_ATTR_DATA2CLOCK_HOLD_TIME", "Descriptive Name"="Data2Clock Hold Time", "Data Type"=1, "Command"="TRIG:SETH:HTIM", "Access"=2, "Range Table"="", "Read Callback"="", "Write Callback"="", "Supported Models"="", "Instrument Options"="", "Flags"=0, "Help"="Sets the minimum time after the clock edge while the data signal must stay steady above or below the data level. The hold time can be negative. In this case, the setup time is always positive. The setup/hold interval starts before the clock edge (setup time) and ends before the clock edge (hold time). If you change the negative hold time, the setup time is adjusted by the intrument.\n\nAvailable Repeated Capabilities:\nNone\n\nRemote-control command(s):\nTRIGger<m>:SETHold:HTIMe"}, {"Level"=3, "Class Only"=FALSE, "Identifier"="RSSCOPE_ATTR_DATA2CLOCK_SETUP_TIME", "Descriptive Name"="Data2Clock Setup Time", "Data Type"=1, "Command"="TRIG:SETH:STIM", "Access"=2, "Range Table"="", "Read Callback"="", "Write Callback"="", "Supported Models"="", "Instrument Options"="", "Flags"=0, "Help"="Sets the minimum time before the clock edge while the data signal must stay steady above or below the data level. The setup time can be negative. In this case, the hold time is always positive. The setup/hold interval starts after the clock edge (setup time) and ends after the clock edge (hold time). If you change the negative setup time, the hold time is adjusted by the intrument.\n\nAvailable Repeated Capabilities:\nNone\n\nRemote-control command(s):\nTRIGger<m>:SETHold:STIMe"}, {"Level"=3, "Class Only"=FALSE, "Identifier"="RSSCOPE_ATTR_DATA2CLOCK_POLARITY", "Descriptive Name"="Data2Clock Polarity", "Data Type"=0, "Command"="TRIG:DAT:CSO:EDGE", "Access"=2, "Range Table"="rsscope_rngPolarity", "Read Callback"="", "Write Callback"="", "Supported Models"="", "Instrument Options"="", "Flags"=0, "Help"="Sets the edge of the clock signal to define the time reference point for the setup and hold time.\n\nAvailable Repeated Capabilities:\nNone\n\nRemote-control command(s):\nTRIGger<m>:DATatoclock:CSOurce:EDGE"}, {"Level"=2, "Class Only"=TRUE, "Identifier"="", "Descriptive Name"="Pattern Triggering", "Data Type"=0, "Command"="", "Access"=0, "Range Table"="", "Read Callback"="", "Write Callback"="", "Supported Models"="", "Instrument Options"="", "Flags"=0, "Help"="The pattern trigger is a logic trigger. It provides logical combinations of the input channels and supports you in verifying the operation of digital logic. The setup of the pattern trigger is very similar to trigger qualification. In addition to the pattern and the trigger levels, you can define a timing condition.\n\nThe pattern trigger is only available for the A-event (Suffix = 1)."}, {"Level"=3, "Class Only"=FALSE, "Identifier"="RSSCOPE_ATTR_PATTERN_MODE", "Descriptive Name"="Pattern Mode", "Data Type"=0, "Command"="TRIG:PATT:MODE", "Access"=2, "Range Table"="rsscope_rngPatternMode", "Read Callback"="", "Write Callback"="", 
